vi "UE9 Config IP Address.vi"() -> ()   [LabVIEW 2021]
panel:
  in  "ConnectionType":string="LJ_ctUSB"
  out "IP Address Read":string="192.168.1.209"
  in  "New IP Address":string="192.168.1.209"
  in  "FirstFound":bool=TRUE
  in  "Address":string="192.168.1.209"
  out "Error Message":string
  in  "error in":errorcluster
  out "error out":errorcluster
  # "Specify an IP address for Ethernet, or Local ID\nfor USB.  If FirstFound is selected, Local ID is\nignored for USB."
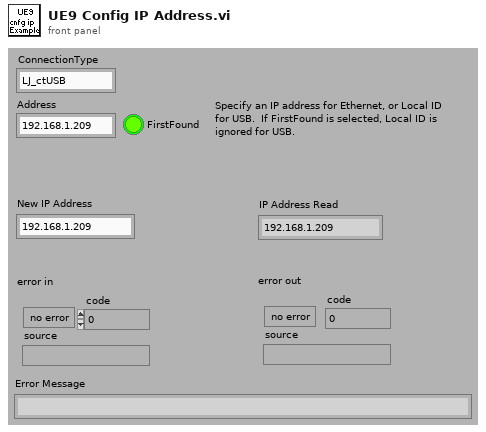
[diagram p1: front panel]
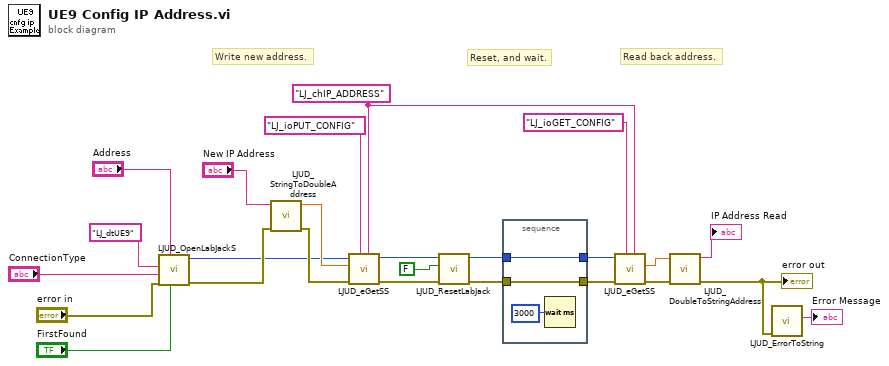
[diagram p0: block diagram]
diagram:
  w16 = "LJ_chIP_ADDRESS" ("Channel")
  # "Read back address."
  # "Reset, and wait."
  # "Write new address."
  n1 = call "LJUD_OpenLabJackS.vi"("FirstFound"="FirstFound", "Address"="Address", "error in"="error in", "ConnectionType"="ConnectionType", "DeviceType"="LJ_dtUE9") -> ("error out"=w4:errorcluster, "Handle"=w3:i32)  [unwired: 4 in, 1 out]
  n2 = call "LJUD_StringToDoubleAddress.vi"("error in"=w4, "String"="New IP Address") -> ("error out"=w22:errorcluster, "Double Address"=w20:dbl)  [unwired: 8 in]
  n3 = call "LJUD_eGetSS.vi"("Channel"=w16, "IOType"="LJ_ioPUT_CONFIG", "error in"=w22, "Value Write"=w20, "Handle In"=w3) -> ("error out"=w18:errorcluster, "Handle Out"=w17:i32)  [unwired: 4 in, 1 out]
  n4 = call "LJUD_ResetLabJack.vi"("error in"=w18, "Soft Reset Only"=FALSE, "Handle In"=w17) -> ("error out"=w13:errorcluster, "Handle Out"=w14:i32)  [unwired: 7 in]
  n5 = stacked-sequence {
    tunnel: w14 -> [w28]
    tunnel: w13 -> [w27]
    tunnel: [w28] -> w12
    tunnel: [w27] -> w11
    frame #0 {
      n6 = Wait (ms)(milliseconds to wait=u32 3000) -> ()  [unwired: 1 out]
    }
  }
  n7 = call "LJUD_eGetSS.vi"("Channel"=w16, "IOType"="LJ_ioGET_CONFIG", "error in"=w11, "Handle In"=w12) -> ("error out"=w10:errorcluster, "Value Read"=w8:dbl)  [unwired: 5 in, 1 out]
  n8 = call "LJUD_DoubleToStringAddress.vi"("error in"=w10, "Double"=w8) -> ("error out"=w9:errorcluster, "String"=→"IP Address Read":string)  [unwired: 8 in]
  "error out" <- w9
  n9 = call "LJUD_ErrorToString.vi"("error in"=w9) -> ("String"=→"Error Message":string)  [unwired: 10 in]
